vi "XY Graph Fold Multiple Plots.vi"(8 "error in (no error)":errorcluster, 9 "# Folds (1)":u32=1, 10 "Selected Plots":i32[](array[numeric]), 11 "Selected Plot Info":T1) -> (0 "error out":errorcluster, 1 "Folded Plot Message":string, 3 "Last Folded Plot":cluster{"t Array":dbl[], "IRF Array":dbl[]}, 4 "Single Plot?":bool)   [LabVIEW 2021, in "XY Graph Add-Ons.lvlib"]
uses:
  XY Graph Add-Ons.lvlib
  XY Graph Selected Plot Info.ctl
  XY Graph Refnum.ctl
  <vilib>/Utility/miscctls.llb/LVPoint32TypeDef.ctl
  Strings/Strings.lvlib
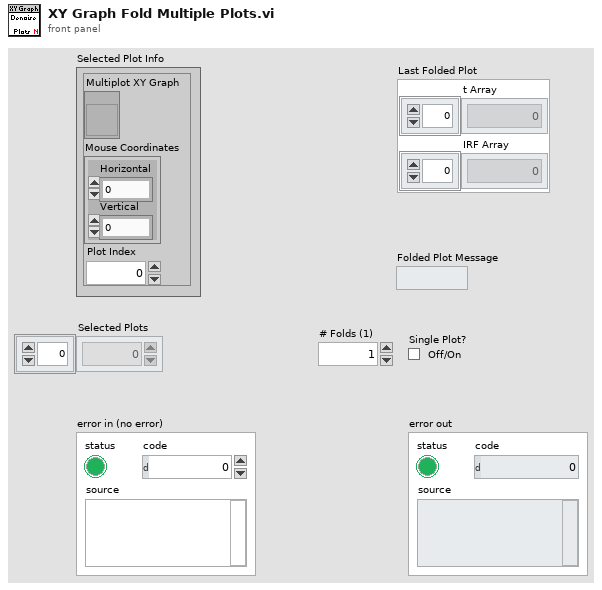
[diagram p1: front panel]
types:
  T1 = typedef "XY Graph Add-Ons.lvlib/XY Graph Selected Plot Info.ctl" = cluster{"Multiplot XY Graph":T2, "Mouse Coordinates":T3, "Plot Index":i32}
  T2 = typedef "XY Graph Add-Ons.lvlib/XY Graph Refnum.ctl" = refnum<vi>
  T3 = typedef "LVPoint32TypeDef.ctl" = cluster{"Horizontal":i32, "Vertical":i32}
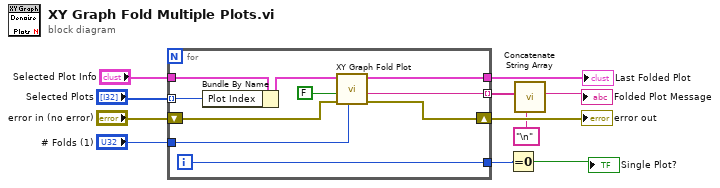
[diagram p0: block diagram]
diagram:
  n1 = for {
    tunnel: "Selected Plot Info" -> [w21]
    tunnel: [w19] -> w6 mode=indexing
    tunnel: [w17] -> w8
    shift-right: [w18] -> w9
    shift-left: "error in (no error)" -> [w20]
    tunnel: "Selected Plots" -> [w15] mode=indexing
    tunnel: [w14] -> w3
    tunnel: "# Folds (1)" -> [w12]
    i -> [w14]
    n2 = Bundle By Name(cluster=w21, "Plot Index"=w15) -> (w16:T1)
    n3 = call "XY Graph Fold Plot.vi"("# Folds (1)"=w12, "error in (no error)"=w20, "Replace Plot (T)?"=FALSE, "Selected Plot Info"=w16) -> ("Error Out"=w18:errorcluster, "Fold Decay Message"=w19:string, "Folded Decay"=w17:cluster{"t Array":dbl[], "IRF Array":dbl[]})  [unwired: 5 in]
  }
  "error out" <- w9
  "Last Folded Plot" <- w8
  n4 = Equal To 0?(x=w3) -> (x = 0?=→"Single Plot?":bool)
  n5 = call "Concatenate String Array.vi"("Separator (TAB)"="\n", "String Array"=w6) -> ("Formatted String"=→"Folded Plot Message":string)  [unwired: 9 in]
